vi "phase_shift.vi"(10 "Numeric":dbl, 11 "waveform":waveform(dbl)) -> (3 "output waveform":waveform(dbl))   [LabVIEW 2015]
uses:
  <vilib>/Analysis/2dsp.llb/Real FFT.vi
  <vilib>/Analysis/2dsp.llb/Inverse Real FFT.vi
  <vilib>/Analysis/NI_AALPro.lvlib
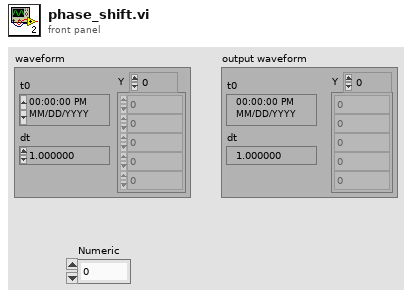
[diagram p1: front panel]
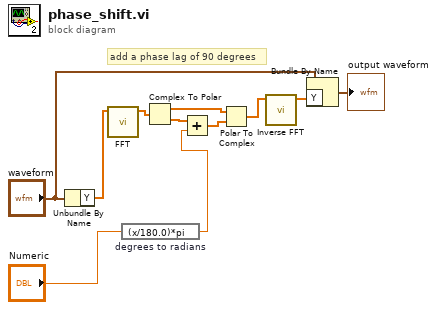
[diagram p0: block diagram]
diagram:
  # "add a phase lag of 90 degrees"
  n1 = Unbundle By Name("waveform") -> ("Y"=w3:dbl[])
  n2 = call-poly <vilib>:"FFT.vi"("X"=w3) -> ("FFT {X}"=w4:cdb[])  [unwired: 9 in, 1 out]
  n3 = expression code="(x/180.0)*pi" "degrees to radians"("Numeric") -> (w2:dbl)
  n4 = Complex To Polar(r * e^(i*theta)=w4) -> (r=w6:dbl[], theta=w5:dbl[])
  n5 = Add(x=w5, y=w2) -> (x+y=w8:dbl[])
  n6 = Polar To Complex(1:w8, 2:w6) -> (0:w7:cdb[])
  n7 = call-poly <vilib>:"Inverse FFT.vi"("FFT {X}"=w7) -> ("X"=w9:dbl[])  [unwired: 9 in, 1 out]
  n8 = Bundle By Name(cluster="waveform", "Y"=w9) -> (→"output waveform":waveform(dbl))
